vi "Autonomous Exec Info.vi"() -> ()   [LabVIEW 2016]
uses:
  Autonomous VIs/Autonomous Commands/Autonomous Command Names.ctl
  Autonomous VIs/Autonomous Exec/Autonomous Play Definition.ctl
panel:
  in  "Command List":cluster{}[](array[cluster])
  in  "Output Play":T1
  out "Autonomous Play\nRead":bool
  in  "Command Information":T3
  out "Number of Commands":dbl
  out "Play Path":path
  out "Play Name":string
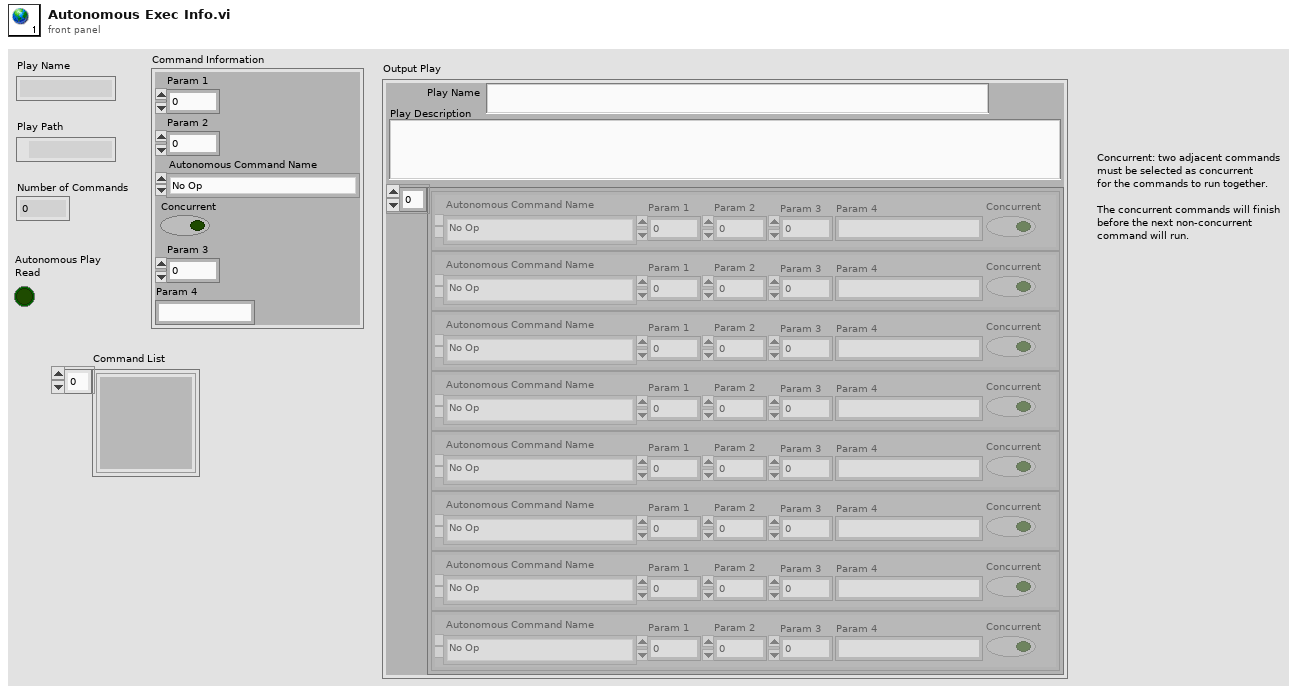
[diagram p1: front panel]
types:
  T1 = typedef "Autonomous Play Definition.ctl" = cluster{"Play Name":string, "Command List":cluster{"Param 1":dbl, "Param 2":dbl, "Autonomous Command Name":T2, "Concurrent":bool, "Param 3":dbl, "Param 4":string}[], "Play Description":string}
  T2 = typedef "Autonomous Command Names.ctl" = enum16{"No Op", "Command Drive+Climb Shift", "Command Wait", "Command Deliver Gear", "Command Buffer", "Command Drive Path", "Command Drive Time", "Command Shoot", "Command Turn to Heading", "Command Run Conveyor", "Command Spinup Shooter", "Command Deliver Gear Front", "Command Toggle Intake Rotation", "DO NOT USE", "Command Agitate Hopper", "Command Pre-Buffer"}
  T3 = cluster{"Param 1":dbl, "Param 2":dbl, "Autonomous Command Name":T2, "Concurrent":bool, "Param 3":dbl, "Param 4":string}
diagram:
